vi "振动判定.vi"(7 "Result":refnum<vi>, 9 "振动判定":T1, 10 "振动判定范围":T2, 11 "FFT":cluster{"f0":dbl, "df":dbl, "magnitude":dbl[]}[](graph)) -> (2 "FFT 2":cluster{"f0":dbl, "df":dbl, "magnitude":dbl[]}[](graph), 3 "OK？":bool)   [LabVIEW 2020]
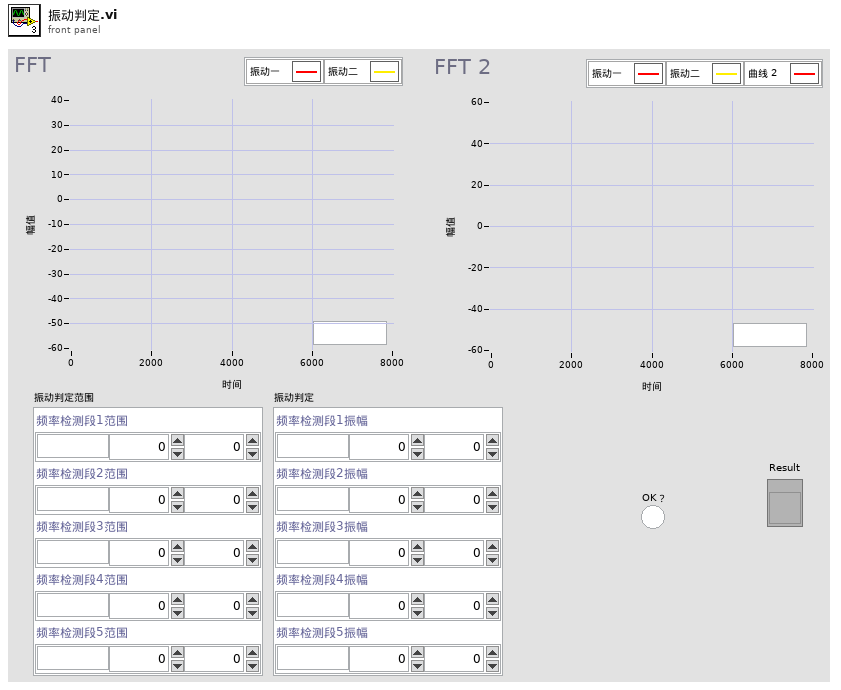
[diagram p1: front panel]
types:
  T1 = cluster{"频率检测段1振幅":cluster{"单位":string, "下限":dbl, "上限":dbl}, "频率检测段2振幅":cluster{"单位":string, "下限":dbl, "上限":dbl}, "频率检测段3振幅":cluster{"单位":string, "下限":dbl, "上限":dbl}, "频率检测段4振幅":cluster{"单位":string, "下限":dbl, "上限":dbl}, "频率检测段5振幅":cluster{"单位":string, "下限":dbl, "上限":dbl}}
  T2 = cluster{"频率检测段1范围":cluster{"单位":string, "下限":dbl, "上限":dbl}, "频率检测段2范围":cluster{"单位":string, "下限":dbl, "上限":dbl}, "频率检测段3范围":cluster{"单位":string, "下限":dbl, "上限":dbl}, "频率检测段4范围":cluster{"单位":string, "下限":dbl, "上限":dbl}, "频率检测段5范围":cluster{"单位":string, "下限":dbl, "上限":dbl}}
  T3 = typedef "svc_Spectrum Info.ctl" = cluster{"channel name":string, "description":string, "x-axis units":T4, "spectral info":cluster{"spectrum type":T5, "linear/dB":enum16{"linear", "dB"}, "window":u16, "window size":i32, "FFT size":i32}, "engineering units":T6, "custom label":string, "dB reference [EU]":dbl, "peak units":enum16{"rms", "peak", "peak-peak"}, "weighting filter":T7, "spectral density?":bool, "unit label":string, "spectrum skewed?":bool, "complimentary spectrum units":T8}
  T4 = typedef "svc_X-Axis Units.ctl" = u16
  T5 = typedef "svc_Spectrum Type.ctl" = enum16{"FFT Spectrum [complex]", "Amplitude [Magnitude]", "Power [Magnitude^2]", "Cross Spectrum [complex]", "Frequency Response [Complex]"}
  T6 = typedef "svc_Engineering Units Text Ring.ctl" = u16
  T7 = typedef "svc_Weighting Filter Text Ring.ctl" = u16
  T8 = typedef "svc_Complimentary Spectrum Units.ctl" = enum16{"none", "radians", "degrees", "cycles", "imaginary"}
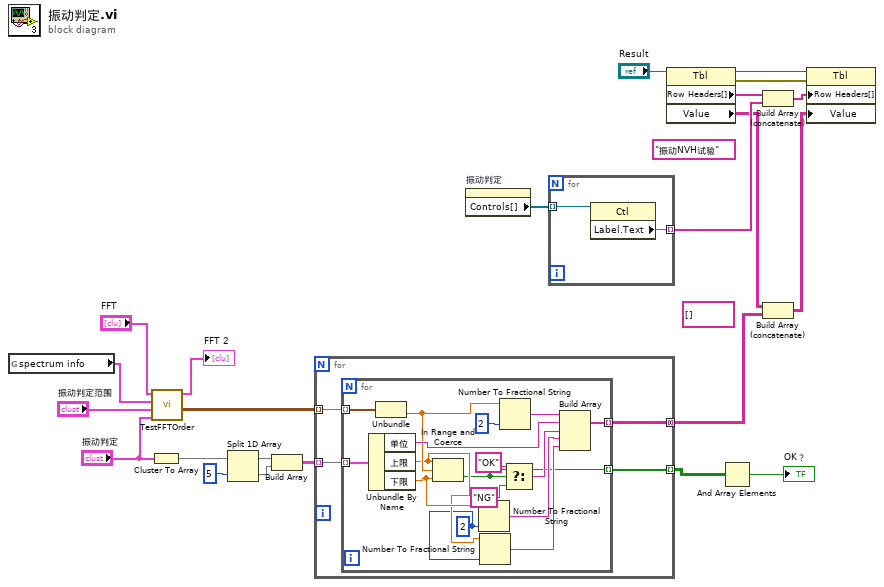
[diagram p0: block diagram]
diagram:
  (unwired) string[] [] ("Label.Text")
  (unwired) "振动NVH试验" ("Label.Text")
  n1 = global read "Global1.vi" "spectrum info"() -> (w22:T3[])
  n2 = Cluster To Array(cluster="振动判定") -> (array=w7:cluster{"单位":string, "下限":dbl, "上限":dbl}[])
  n3 = call "TestFFTOrder.vi"("振动判定"="振动判定", "振动判定范围"="振动判定范围", "spectrum info"=w22, "FFT 5"="FFT") -> ("数组"=w13:cluster{"freq.":dbl, "dB":dbl}[][], "FFT 2"=→"FFT 2":cluster{"x0":dbl, "dx":dbl, "Y":dbl[]}[])  [unwired: 5 in, 1 out]
  n4 = Split 1D Array(array=w7, index=5 ("索引")) -> (first subarray=w6:cluster{"单位":string, "下限":dbl, "上限":dbl}[], second subarray=w5:cluster{"单位":string, "下限":dbl, "上限":dbl}[])
  n5 = Build Array(w6, w5) -> (w4:cluster{"单位":string, "下限":dbl, "上限":dbl}[][])
  n6 = for {
    tunnel: w13 -> [w27] mode=indexing
    tunnel: [w25] -> w2 mode=concatenating
    tunnel: w4 -> [w26] mode=indexing
    tunnel: [w24] -> w1 mode=indexing
    n7 = for {
      tunnel: w27 -> [w43] mode=indexing
      tunnel: w26 -> [w41] mode=indexing
      tunnel: [w36] -> w25 mode=indexing
      tunnel: [w28] -> w24 mode=indexing
      w29 = i16 2 ("精度(6)")
      n8 = Unbundle By Name(w41) -> ("单位"=w38:string, "上限"=w30:dbl, "下限"=w33:dbl)
      n9 = Unbundle(w43) -> ("dB"=w34:dbl)  [unwired: 1 out]
      n10 = In Range and Coerce(upper limit=w30, x=w34, lower limit=w33) -> (In Range?=w28:bool)  [unwired: 1 out]
      n11 = Number To Fractional String(number=w33, precision (6)=w29) -> (F-format string=w32:string)  [unwired: 2 in]
      n12 = Number To Fractional String(number=w30, precision (6)=w29) -> (F-format string=w31:string)  [unwired: 2 in]
      n13 = Number To Fractional String(number=w34, precision (6)=i16 2 ("精度(6)")) -> (F-format string=w37:string)  [unwired: 2 in]
      n14 = Select(t="OK", s=w28, f="NG") -> (s? t:f=w39:string)
      n15 = Build Array(w37, w38, w39, w32, w31) -> (w36:string[])
    }
  }
  n16 = property on="振动判定" class="Clust (严格)"() -> ("Controls[]"=w15:refnum<vi>[])  [unwired: 2 in, 2 out]
  n17 = for {
    tunnel: w15 -> [w45] mode=indexing
    tunnel: [w44] -> w14 mode=indexing
    n18 = property class="Ctl"(reference=w45) -> ("Label.Text"=w44:string)  [unwired: 1 in, 2 out]
  }
  n19 = property class="Tbl"(reference="Result") -> (reference out=w19:refnum<vi>, error out=w20:errorcluster, "Row Headers[]"=w16:string[], "Value"=w12:string[][])  [unwired: 1 in]
  n20 = And Array Elements(Boolean array=w1) -> (logical AND=→"OK？":bool)
  n21 = Build Array (concatenate)(w16, w14) -> (w18:string[])
  n22 = Build Array (concatenate)(w12, w2) -> (w11:string[][])
  n23 = property class="Tbl"(reference=w19, error in=w20, "Row Headers[]"=w18, "Value"=w11) -> ()  [unwired: 2 out]
